vi "Clear Sweeps.vi"(11 "error in (no error)":errorcluster) -> (15 "error out":errorcluster)   [LabVIEW 2023, in "RFCalAndFixtureCharact.Common.lvlib"]
uses:
  RFCalAndFixtureCharact.Common.lvlib
  Type Definitions/Dictionary Operation.ctl
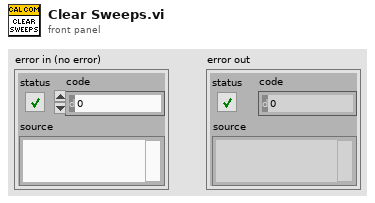
[diagram p1: front panel]
types:
  T1 = typedef "RFCalAndFixtureCharact.Common.lvlib/Dictionary Operation.ctl" = enum16{"Read", "Insert", "Remove", "Clear", "Get All", "Update"}
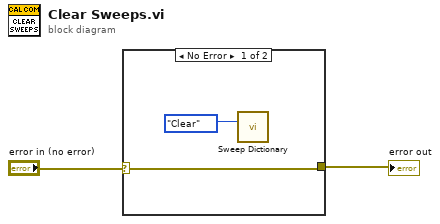
[diagram p0: block diagram]
diagram:
  n1 = case shown="No Error" "error in (no error)" {
    selector: "error in (no error)" -> [w3 w5]
    tunnel: [w3 w5] -> w1
    frame No Error {
      n2 = call "Sweep Dictionary.vi"("Action"=Dictionary_Operation."Clear") -> ()  [unwired: 12 in, 3 out]
    }
    frame Error {
    }
  }
  "error out" <- w1
